vi "set initial zoom.vi"(9 "reset?":bool, 10 "Image Refs In":T1[](array[typedef]), 11 "DisplayRefsIn(generic class)":refnum<vi>[](array[refnum])) -> ()   [LabVIEW 2012]
uses:
  <vilib>/vision/Image Controls.llb/IMAQ Image.ctl
panel:
  out "VI name":string
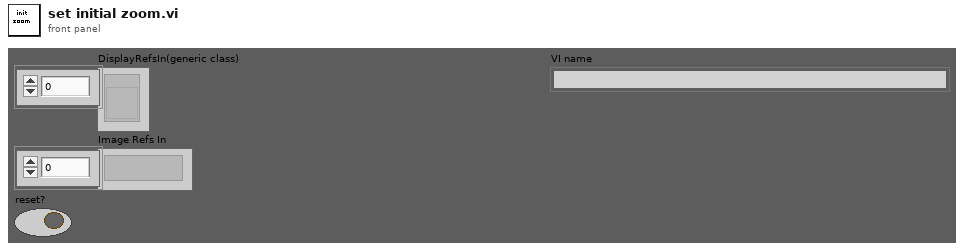
[diagram p1: front panel]
types:
  T1 = typedef "IMAQ Image.ctl" = refnum<image>
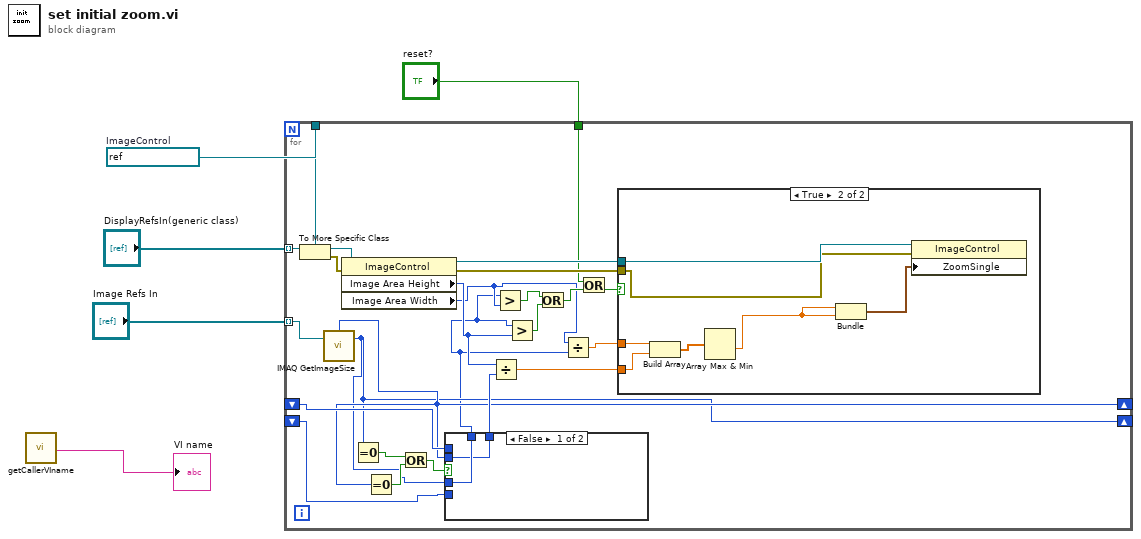
[diagram p0: block diagram]
diagram:
  w5 = refnum<vi> refnum  # ImageControl
  n1 = call "getCallerVIname.vi"() -> ("VI name"=→"VI name":string)  [unwired: 19 in]
  n2 = for {
    tunnel: w5 -> [w30]
    tunnel: "DisplayRefsIn(generic class)" -> [w29] mode=indexing
    tunnel: "Image Refs In" -> [w24] mode=indexing
    tunnel: "reset?" -> [w17]
    shift-right: [w7] -> _
    shift-left: _ -> [w10]
    shift-right: [w8] -> _
    shift-left: _ -> [w11]
    n3 = To More Specific Class(target class=w30, reference=w29) -> (specific class reference=w28:refnum<vi>, error out=w25:errorcluster)  [unwired: 1 in]
    n4 = call "IMAQ GetImageSize"("Image"=w24) -> ("Y Resolution"=w7:i32, "X Resolution"=w8:i32)  [unwired: 3 in, 1 out]
    n5 = property class="ImageControl"(reference=w28, error in=w25) -> (reference out=w27:refnum<vi>, error out=w26:errorcluster, "Image Area Height"=w16:u32, "Image Area Width"=w15:u32)
    n6 = Equal To 0?(x=w7) -> (x = 0?=w14:bool)
    n7 = Equal To 0?(x=w8) -> (x = 0?=w13:bool)
    n8 = Or(x=w14, y=w13) -> (x .or. y?=w12:bool)
    n9 = case shown="False" w12 {
      tunnel: w11 -> [_ w34]
      tunnel: w10 -> [_ w33]
      tunnel: [w31 w34] -> w9
      tunnel: w8 -> [w31 _]
      tunnel: [w32 w33] -> w6
      tunnel: w7 -> [w32 _]
      frame False {
      }
      frame True {
      }
    }
    n10 = Divide(x=w16, y=w9) -> (x/y=w20:dbl)
    n11 = Greater?(x=w6, y=w15) -> (0:w23:bool)
    n12 = Greater?(x=w6, y=w16) -> (0:w22:bool)
    n13 = Or(x=w23, y=w22) -> (x .or. y?=w21:bool)
    n14 = Divide(x=w15, y=w6) -> (x/y=w19:dbl)
    n15 = Or(x=w17, y=w21) -> (x .or. y?=w18:bool)
    n16 = case shown="True" w18 {
      tunnel: w27 -> [_ w41]
      tunnel: w26 -> [_ w40]
      tunnel: w20 -> [_ w37]
      tunnel: w19 -> [_ w38]
      frame False {
      }
      frame True {
        n17 = Build Array(w38, w37) -> (w36:dbl[])
        n18 = Array Max & Min(array=w36) -> (min value=w35:dbl)  [unwired: 3 out]
        n19 = Bundle(w35, w35) -> (w39:cluster{dbl, dbl})  [unwired: 1 in]
        n20 = property class="ImageControl"(reference=w41, error in=w40, "ZoomSingle"=w39) -> ()  [unwired: 2 out]
      }
    }
  }
